vi "Update Price Schedule.vi"(10 "Price Schedule":T1, 11 "Optimization in":refnum<class "Optimization.lvclass">) -> (3 "Optimization out":refnum<class "Optimization.lvclass">)   [LabVIEW 2016, in "Optimization Framework.lvlib" / "Optimization.lvclass"]
uses:
  Optimization.lvclass
  Controls/Schedule Price.ctl
  Optimization.lvclass/Optimization.ctl
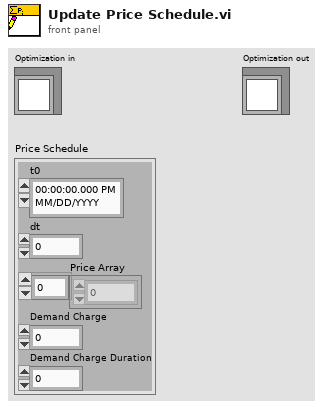
[diagram p1: front panel]
types:
  T1 = typedef "Optimization Framework.lvlib/Optimization.lvclass/Schedule Price.ctl" = cluster{"t0":timestamp, "dt":dbl, "Price Array":dbl[], "Demand Charge":dbl, "Demand Charge Duration":dbl}
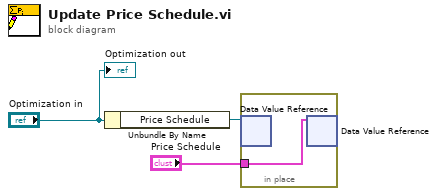
[diagram p0: block diagram]
diagram:
  n1 = Unbundle By Name("Optimization in") -> ("Price Schedule"=w3:refnum<data-value>)
  n2 = in-place {
    in-place-border: "Price Schedule" -> [w4]
    n3 = in-place-dvr #1(w3) -> ()  [unwired: 2 out]
    n4 = in-place-dvr #1(w4) -> ()  [unwired: 2 out]
  }
  "Optimization out" <- "Optimization in"
